vi "Make Default QPS.vi"() -> (3 "QPS settings":T1={"TWM pipe name"="", "meas"={"Measurement ID"=enum."Manual setup", "Description"="", "Switching matrix M"=[], "Signal frequency  (Hz)"=0.0, "Maximal signal amplitude (V)"=0.0, "PRs (samples)"=0, "PRe (samples)"=0, "MRs (samples)"=0, "MRe (samples)"=0, "Set PJVS frequency (Hz)"=0.0, "PJVS reference voltages (1 period, V)"=[], "Requiested PJVS steps"=0, "Sampling f (Hz)"=0.0, "Trigger mode"=enum."Trigger every MX switch", "Timing matrix (periods)"=[], "Record length (multiples of M)"=0, "Calculated"={"Triggers to next path (line of sequence)"=[], "Record samples"=0, "Sample indexes of switches"=[], "PRs (s)"=5.0, "PRe (s)"=5.0, "MRs (s)"=0.0, "MRe (s)"=0.0, "Trigger frequency  (Hz)"=0.0, "Measurement druation (s)"=0.0, "Samples per step"=0.0, "QPMX Sequence"=[], "PJVS segments frequency (Hz)"=50.0}, "No of required digitizers"=0, "No of required transducers"=0, "Transducer correction files"=[], "Digitizer correction file"=path "", "Algorithm"="TWM-PWRFFT", "plots_level"=1}, "PJVS setup"={"PJVS type"=enum."AC-supraVOLTcontrol", "Status Refnum"=refnum, "AC-supraVOLTcontrol"={"IP address:port (0.0.0.0:0000)"="", "Timeouts"={"TCP Read & Write (ms)"=0, "Sensors readout"=0, "PJVS setup"=0, "Nullmeter readout"=0, "Multiplexer setup"=0, "57XX setup"=0, "Generator setup"=0, "Synthesizer setup"=0, "Sampler readout"=0}, "Simulation mode"=FALSE, "Debug mode"=FALSE}, "NPL bias source"={"DataSocketCluster"={"Server Machine"="", "Client Machine"="", "Data"="", "TimeStamp"=0.0, "Count"=0, "Target Process"=""}}, "Manual PJVS"={"PJVS frequency (Hz)"=0.0, "Reference voltages (V)"=[], "File with PJVS voltages"=path ""}, "VTT PJVS"={"some VTT only property"=""}}, "Measurement status Ref"=refnum, "TWM status Ref"=refnum, "Abort Ref"=refnum, "AWG"={"AWG type"=enum."Agilent 331xxA to 332xxA", "FGEN Resource Name"="", "Source (Onboard Clock)"="", "FGEN Channel"="", "awg lib session"={"type"=enum."Agilent 331xxA to 332xxA", "VISA"="", "enable 10MHz ref"=FALSE, "cmi ckd2"={"VISA"="", "clock source"=enum."Auto", "manual ref clk"=FALSE, "ref clock [Hz]"=0.0, "div mode"=enum."Set divisor directly"}, "cmi sync v3"={"VISA"="", "baud rate [bd/s]"=0, "source"=enum."Auto", "hv range"=enum."10V", "fsrc is fixed"=FALSE, "fsrc [Hz]"=0.0, "freq integ [s]"=0.0, "freq filter"=0, "trig level"=enum."LVCMOS 3V3", "chn1 mode"=enum."Source divider", "chn1 level"=enum."Positive 3V3", "chn2 mode"=enum."Source divider", "chn2 level"=enum."Positive 3V3", "chn2 div"=0, "chn3 mode"=enum."Chn 1 Active", "chn3 level"=enum."Positive 3V3", "chn1 div entry"=enum."Set divisor directly", "chn1 dev limit [%]"=0.0, "chn1 check dev"=FALSE}, "trigger"={"source"=enum."Immediate", "level [V]"=0.0, "coupling"=enum."DC", "slope"=enum."POS"}, "HMF2500 cfg"={"Baud Rate"=0, "Parity"=0, "Data Bits"=0, "Flow Control"=0}}}} {"AWG"."awg lib session"."HMF2500 cfg"."Flow Control" items=["None", "XON/XOFF", "RTS/CTS", "XON/XOFF & RTS/CTS", "DTR/DSR", "XON/XOFF & DTR/DSR"]; "AWG"."awg lib session"."HMF2500 cfg"."Data Bits" items=["7"=7, "8"=8]; "AWG"."awg lib session"."HMF2500 cfg"."Parity" items=["None", "Odd", "Even", "Mark", "Space"]; "AWG"."awg lib session"."HMF2500 cfg"."Baud Rate" items=["300"=300, "600"=600, "1200"=1200, "2400"=2400, "4800"=4800, "9600"=9600, "19200"=19200]; "AWG"."awg lib session"."cmi sync v3"."chn2 div" min=1 max=100000000 step=1; "AWG"."awg lib session"."cmi sync v3"."fsrc [Hz]" format="%_8p"; "PJVS setup"."NPL bias source"."DataSocketCluster"."TimeStamp" format="%.2f"; "meas"."plots_level" max=4 step=1; "meas"."Calculated"."Trigger frequency  (Hz)" format="%#_6p"; "meas"."Record length (multiples of M)" min=1 step=1; "meas"."PJVS reference voltages (1 period, V)" format="%.9g"})   [LabVIEW 2020]
doc: "Returns QPS set to default values."
uses:
  General PJVS driver/QPSsettings.ctl
  Measurement/Type definitions/Measuement properties.ctl
  Measurement/Type definitions/Measurement ID.ctl
  Measurement/Type definitions/Trigger mode.ctl
  General PJVS driver/Type definitions/PJVS Setup.ctl
  General PJVS driver/Type definitions/PJVS Type.ctl
  PJVS drivers/acsvcontrol-driver/build/ACSVcontrol-driver_0.2.1.0.llb/Timeouts.ctl
  PJVS drivers/JV modified NPL Bias source/DataSocketCluster external.ctl
  General AWG/Type definitions/AWG.ctl
  General AWG/Type definitions/AWG type.ctl
  <instrlib>/niFgen/niFgen.llb/niFgen_ctl Sample Clock Source Values (Ring).ctl
  external libraries/AWG/AWG Session.ctl
  external libraries/AWG/AWG Type.ctl
  external libraries/AWG/CMI Clock Divider v2/CMI ckd2 Session.ctl
  external libraries/AWG/CMI Clock Divider v2/CMI ckd2 Source Mode.ctl
  external libraries/AWG/CMI Clock Divider v2/CMI ckd2 Divisor Mode.ctl
  external libraries/AWG/CMI Sync V3/CMI Sync V3 session.ctl
  external libraries/AWG/CMI Sync V3/Configure/CMI Sync V3 Reference Clock Source.ctl
  external libraries/AWG/CMI Sync V3/Configure/CMI Sync V3 HV input Range.ctl
  external libraries/AWG/CMI Sync V3/Configure/CMI Sync V3 Trigger Input Level.ctl
  external libraries/AWG/CMI Sync V3/Configure/CMI Sync V3 Channel 1 Mode.ctl
  external libraries/AWG/CMI Sync V3/Configure/CMI Sync V3 Channel Output Levels.ctl
  external libraries/AWG/CMI Sync V3/Configure/CMI Sync V3 Channel 2 Mode.ctl
  external libraries/AWG/CMI Sync V3/Configure/CMI Sync V3 Channel 3 Mode.ctl
  external libraries/AWG/CMI Sync V3/Configure/CMI Sync V3 Channel 1 Divisor Entry Mode.ctl
  external libraries/externals needed for AWG/ADC Trig Config.ctl
  external libraries/externals needed for AWG/ADC Trig Mode Source.ctl
  external libraries/externals needed for AWG/ADC Trig Coupling.ctl
  external libraries/externals needed for AWG/ADC Trig Slope.ctl
  external libraries/AWG/RaS HMF2500/HMF2500 Config.ctl
  external libraries/AWG/AWG.lvlib
  external libraries/AWG/CMI Sync V3/CMI Sync Unit V3.lvlib
  PJVS drivers/acsvcontrol-driver/build/ACSVcontrol-driver_0.2.1.0.llb/ACSVcontrol-driver.lvlib
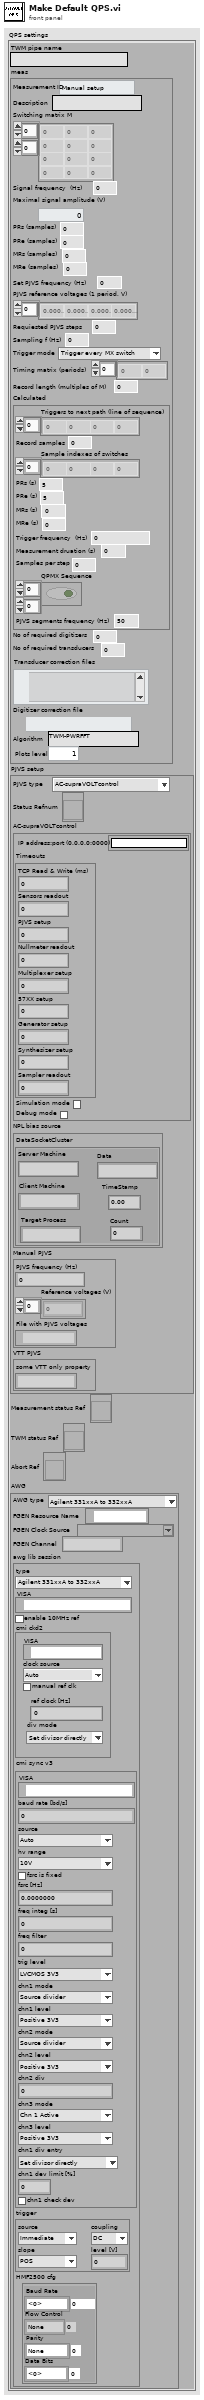
[diagram p1: front panel]
types:
  T1 = typedef "QPSsettings.ctl" = cluster{"TWM pipe name":string, "meas":T2, "PJVS setup":T5, "Measurement status Ref":refnum<vi>, "TWM status Ref":refnum<vi>, "Abort Ref":refnum<vi>, "AWG":T9}
  T2 = typedef "Measuement properties.ctl" = cluster{"Measurement ID":T3, "Description":string, "Switching matrix M":i32[][], "Signal frequency  (Hz)":dbl, "Maximal signal amplitude (V)":dbl, "PRs (samples)":u32, "PRe (samples)":u32, "MRs (samples)":u32, "MRe (samples)":u32, "Set PJVS frequency (Hz)":dbl, "PJVS reference voltages (1 period, V)":dbl[], "Requiested PJVS steps":u32, "Sampling f (Hz)":dbl, "Trigger mode":T4, "Timing matrix (periods)":i32[], "Record length (multiples of M)":u32, "Calculated":cluster{"Triggers to next path (line of sequence)":u32[], "Record samples":u32, "Sample indexes of switches":u32[], "PRs (s)":dbl, "PRe (s)":dbl, "MRs (s)":dbl, "MRe (s)":dbl, "Trigger frequency  (Hz)":dbl, "Measurement druation (s)":dbl, "Samples per step":dbl, "QPMX Sequence":bool[][], "PJVS segments frequency (Hz)":dbl}, "No of required digitizers":u32, "No of required transducers":u32, "Transducer correction files":path[], "Digitizer correction file":path, "Algorithm":string, "plots_level":u32}
  T3 = typedef "Measurement ID.ctl" = enum16{"Manual setup", "1 signal, 1 ADC, 1 PJVS", "1 phase (U, I), 1 ADC, 1 PJVS", "1 phase (U, I), 2 ADC, 1 PJVS", "1 phase (U, I), 3 ADC, 1 PJVS", "3 phases (U1..3, I1..3), 3 ADC, 1 PJVS"}
  T4 = typedef "Trigger mode.ctl" = enum16{"Trigger every MX switch", "Trigger every sample"}
  T5 = typedef "PJVS Setup.ctl" = cluster{"PJVS type":T6, "Status Refnum":refnum<vi>, "AC-supraVOLTcontrol":cluster{"IP address:port (0.0.0.0:0000)":string, "Timeouts":T7, "Simulation mode":bool, "Debug mode":bool}, "NPL bias source":cluster{"DataSocketCluster":T8}, "Manual PJVS":cluster{"PJVS frequency (Hz)":dbl, "Reference voltages (V)":dbl[], "File with PJVS voltages":path}, "VTT PJVS":cluster{"some VTT only property":string}}
  T6 = typedef "PJVS Type.ctl" = enum16{"AC-supraVOLTcontrol", "JV modified NPL bias control", "Manual PJVS", "VTT PJVS"}
  T7 = typedef "ACSVcontrol-driver.lvlib/Timeouts.ctl" = cluster{"TCP Read & Write (ms)":i32, "Sensors readout":i32, "PJVS setup":i32, "Nullmeter readout":i32, "Multiplexer setup":i32, "57XX setup":i32, "Generator setup":i32, "Synthesizer setup":i32, "Sampler readout":i32}
  T8 = typedef "DataSocketCluster external.ctl" = cluster{"Server Machine":string, "Client Machine":string, "Data":string, "TimeStamp":dbl, "Count":i32, "Target Process":string}
  T9 = typedef "AWG.ctl" = cluster{"AWG type":T10, "FGEN Resource Name":refnum<k15>, "Source (Onboard Clock)":T11, "FGEN Channel":string, "awg lib session":T12}
  T10 = typedef "AWG type.ctl" = enum16{"Agilent 331xxA to 332xxA", "Agilent 335xxA to 336xxA", "Tektronix AFG3101C", "R&S HMF25xx", "CMI Clock Divider v2", "CMI Sync Unit V3", "FGEN NI 5413", "Supracon PJVS Generator", "dummy"}
  T11 = typedef "niFgen_ctl Sample Clock Source Values (Ring).ctl" = string
  T12 = typedef "AWG.lvlib/AWG Session.ctl" = cluster{"type":T13, "VISA":refnum<visa-resource-name>, "enable 10MHz ref":bool, "cmi ckd2":T14, "cmi sync v3":T17, "trigger":T26, "HMF2500 cfg":T30}
  T13 = typedef "AWG.lvlib/AWG Type.ctl" = enum16{"Agilent 331xxA to 332xxA", "Agilent 335xxA to 336xxA", "Tektronix AFG3101C", "R&S HMF25xx", "CMI Clock Divider v2", "CMI Sync Unit V3", "dummy"}
  T14 = typedef "AWG.lvlib/CMI ckd2 Session.ctl" = cluster{"VISA":refnum<visa-resource-name>, "clock source":T15, "manual ref clk":bool, "ref clock [Hz]":dbl, "div mode":T16}
  T15 = typedef "AWG.lvlib/CMI ckd2 Source Mode.ctl" = enum16{"Auto", "LF clock", "HF clock", "Internal"}
  T16 = typedef "AWG.lvlib/CMI ckd2 Divisor Mode.ctl" = enum16{"Set divisor directly", "Set divisor by frequency"}
  T17 = typedef "AWG.lvlib/CMI Sync Unit V3.lvlib/CMI Sync V3 session.ctl" = cluster{"VISA":refnum<visa-resource-name>, "baud rate [bd/s]":i32, "source":T18, "hv range":T19, "fsrc is fixed":bool, "fsrc [Hz]":dbl, "freq integ [s]":dbl, "freq filter":i32, "trig level":T20, "chn1 mode":T21, "chn1 level":T22, "chn2 mode":T23, "chn2 level":T22, "chn2 div":i32, "chn3 mode":T24, "chn3 level":T22, "chn1 div entry":T25, "chn1 dev limit [%]":dbl, "chn1 check dev":bool}
  T18 = typedef "AWG.lvlib/CMI Sync Unit V3.lvlib/CMI Sync V3 Reference Clock Source.ctl" = enum16{"Auto", "Internal", "Logic", "Sine", "HV"}
  T19 = typedef "AWG.lvlib/CMI Sync Unit V3.lvlib/CMI Sync V3 HV input Range.ctl" = enum16{"10V", "60V", "250V", "1kV"}
  T20 = typedef "AWG.lvlib/CMI Sync Unit V3.lvlib/CMI Sync V3 Trigger Input Level.ctl" = enum16{"LVCMOS 3V3", "TTL 5V"}
  T21 = typedef "AWG.lvlib/CMI Sync Unit V3.lvlib/CMI Sync V3 Channel 1 Mode.ctl" = enum16{"Source divider", "DDS absolute", "DDS ratio", "DDS ratio M/N"}
  T22 = typedef "AWG.lvlib/CMI Sync Unit V3.lvlib/CMI Sync V3 Channel Output Levels.ctl" = enum16{"Positive 3V3", "Negative 3V3", "Positive 5V", "Negative 5V"}
  T23 = typedef "AWG.lvlib/CMI Sync Unit V3.lvlib/CMI Sync V3 Channel 2 Mode.ctl" = enum16{"Source divider", "Chn 1 divide"}
  T24 = typedef "AWG.lvlib/CMI Sync Unit V3.lvlib/CMI Sync V3 Channel 3 Mode.ctl" = enum16{"Chn 1 Active", "Chn 2 Active", "Chn 1 Trigger", "Chn 2 Trigger", "Gate", "PPS", "10MHz"}
  T25 = typedef "AWG.lvlib/CMI Sync Unit V3.lvlib/CMI Sync V3 Channel 1 Divisor Entry Mode.ctl" = enum16{"Set divisor directly", "Calculate nearest divisor from measured fx"}
  T26 = typedef "ADC Trig Config.ctl" = cluster{"source":T27, "level [V]":dbl, "coupling":T28, "slope":T29}
  T27 = typedef "ADC Trig Mode Source.ctl" = enum16{"Immediate", "External", "Level"}
  T28 = typedef "ADC Trig Coupling.ctl" = enum16{"DC", "AC"}
  T29 = typedef "ADC Trig Slope.ctl" = enum16{"POS", "NEG"}
  T30 = typedef "AWG.lvlib/HMF2500 Config.ctl" = cluster{"Baud Rate":u32, "Parity":u16, "Data Bits":u16, "Flow Control":u16}
  T31 = cluster{"Triggers to next path (line of sequence)":u32[], "Record samples":u32, "Sample indexes of switches":u32[], "PRs (s)":dbl, "PRe (s)":dbl, "MRs (s)":dbl, "MRe (s)":dbl, "Trigger frequency  (Hz)":dbl, "Measurement druation (s)":dbl, "Samples per step":dbl, "QPMX Sequence":bool[][], "PJVS segments frequency (Hz)":dbl}
  T32 = cluster{"PJVS frequency (Hz)":dbl, "Reference voltages (V)":dbl[], "File with PJVS voltages":path}
  T33 = cluster{"IP address:port (0.0.0.0:0000)":string, "Timeouts":T7, "Simulation mode":bool, "Debug mode":bool}
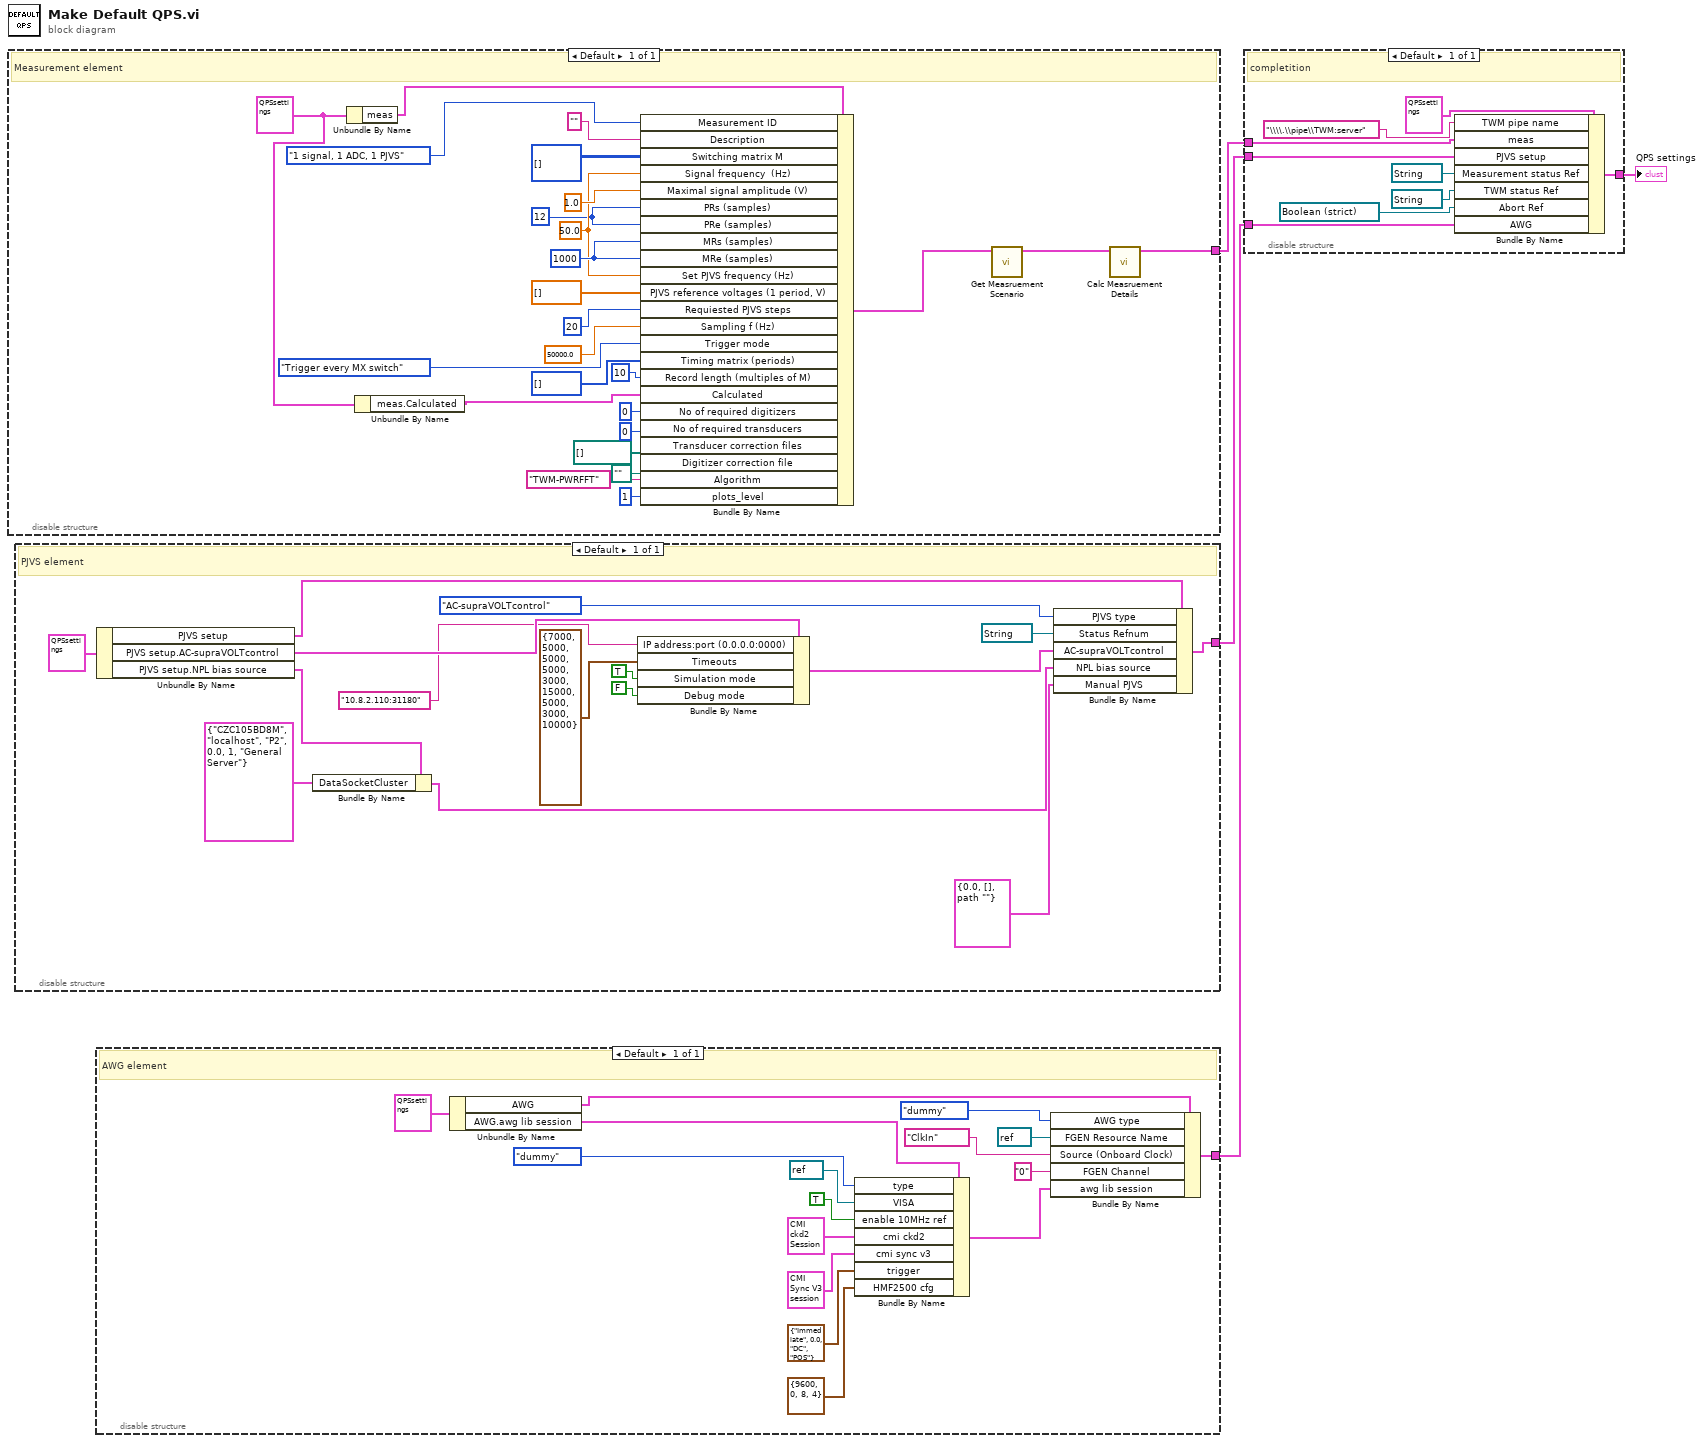
[diagram p0: block diagram]
diagram:
  n1 = disable-structure shown="Default" {
    disable-tunnel: [w16] -> w3
    frame Enabled {
      w7 = u32 12 ("Signal frequency  (Hz)")
      w9 = T1 {"TWM pipe name"="\\\\.\\pipe\\TWM:server", "meas"={"Measurement ID"=enum."1 signal, 1 ADC, 1 PJVS", "Description"="3 phase, 3 ADC, 1 PJVS", "Switching matrix M"=[], "Signal frequency  (Hz)"=50.0, "Maximal signal amplitude (V)"=0.0, "PRs (samples)"=1, "PRe (samples)"=10, "MRs (samples)"=0, "MRe (samples)"=0, "Set PJVS frequency (Hz)"=50.0, "PJVS reference voltages (1 period, V)"=[], "Requiested PJVS steps"=10, "Sampling f (Hz)"=7000.0, "Trigger mode"=enum."Trigger every MX switch", "Timing matrix (periods)"=[], "Record length (multiples of M)"=1, "Calculated"={"Triggers to next path (line of sequence)"=[], "Record samples"=0, "Sample indexes of switches"=[], "PRs (s)"=0.0, "PRe (s)"=0.0, "MRs (s)"=0.0, "MRe (s)"=0.0, "Trigger frequency  (Hz)"=50.0, "Measurement druation (s)"=0.0, "Samples per step"=0.0, "QPMX Sequence"=[], "PJVS segments frequency (Hz)"=50.0}, "No of required digitizers"=0, "No of required transducers"=0, "Transducer correction files"=[], "Digitizer correction file"=path "", "Algorithm"="TWM-PWRFFT", "plots_level"=1}, "PJVS setup"={"PJVS type"=enum."AC-supraVOLTcontrol", "Status Refnum"=refnum, "AC-supraVOLTcontrol"={"IP address:port (0.0.0.0:0000)"="0.0.0.0:0000", "Timeouts"={"TCP Read & Write (ms)"=7000, "Sensors readout"=5000, "PJVS setup"=10000, "Nullmeter readout"=5000, "Multiplexer setup"=3000, "57XX setup"=15000, "Generator setup"=5000, "Synthesizer setup"=3000, "Sampler readout"=10000}, "Simulation mode"=FALSE, "Debug mode"=FALSE}, "NPL bias source"={"DataSocketCluster"={"Server Machine"="CZC105BD8M", "Client Machine"="localhost", "Data"="P2", "TimeStamp"=0.0, "Count"=1, "Target Process"="General Server"}}, "Manual PJVS"={"PJVS frequency (Hz)"=0.0, "Reference voltages (V)"=[], "File with PJVS voltages"=path ""}, "VTT PJVS"={"some VTT only property"=""}}, "Measurement status Ref"=refnum, "TWM status Ref"=refnum, "Abort Ref"=refnum, "AWG"={"AWG type"=enum."Agilent 331xxA to 332xxA", "FGEN Resource Name"="", "Source (Onboard Clock)"="OnboardClock", "FGEN Channel"="0", "awg lib session"={"type"=enum."Agilent 331xxA to 332xxA", "VISA"="", "enable 10MHz ref"=FALSE, "cmi ckd2"={"VISA"="", "clock source"=enum."Auto", "manual ref clk"=FALSE, "ref clock [Hz]"=0.0, "div mode"=enum."Set divisor directly"}, "cmi sync v3"={"VISA"="", "baud rate [bd/s]"=115200, "source"=enum."Auto", "hv range"=enum."1kV", "fsrc is fixed"=FALSE, "fsrc [Hz]"=10000000.0, "freq integ [s]"=1.0, "freq filter"=5, "trig level"=enum."TTL 5V", "chn1 mode"=enum."Source divider", "chn1 level"=enum."Positive 5V", "chn2 mode"=enum."Source divider", "chn2 level"=enum."Positive 5V", "chn2 div"=1, "chn3 mode"=enum."Chn 1 Active", "chn3 level"=enum."Positive 5V", "chn1 div entry"=enum."Calculate nearest divisor from measured fx", "chn1 dev limit [%]"=1.0, "chn1 check dev"=FALSE}, "trigger"={"source"=enum."Immediate", "level [V]"=0.0, "coupling"=enum."DC", "slope"=enum."POS"}, "HMF2500 cfg"={"Baud Rate"=9600, "Parity"=0, "Data Bits"=8, "Flow Control"=4}}}} ("QPS settings")
      w25 = u32 1000 ("PRs (s)")
      w24 = 50.0 ("Signal frequency  (Hz)")
      # "Measurement element"
      n2 = Unbundle By Name(w9) -> ("meas"=w29:T2)
      n3 = Unbundle By Name(w9) -> ("meas.Calculated"=w8:T31)
      n4 = Bundle By Name(cluster=w29, "Measurement ID"=Measurement_ID."1 signal, 1 ADC, 1 PJVS", "Description"="", "Switching matrix M"=u32[][] [], "Signal frequency  (Hz)"=w24, "Maximal signal amplitude (V)"=1.0, "PRs (samples)"=w7, "PRe (samples)"=w7, "MRs (samples)"=w25, "MRe (samples)"=w25, "Set PJVS frequency (Hz)"=w24, "PJVS reference voltages (1 period, V)"=dbl[] [], "Requiested PJVS steps"=u32 20, "Sampling f (Hz)"=50000.0, "Trigger mode"=Trigger_mode."Trigger every MX switch", "Timing matrix (periods)"=i32[] [], "Record length (multiples of M)"=u32 10, "Calculated"=w8, "No of required digitizers"=u32 0, "No of required transducers"=u32 0, "Transducer correction files"=path[] [], "Digitizer correction file"=path "", "Algorithm"="TWM-PWRFFT", "plots_level"=u32 1) -> (w17:T2)
      n5 = call "Get Measruement Scenario.vi"("Measurement properties"=w17) -> ("Measurement properties out"=w27:T2)  [unwired: 10 in]
      n6 = call "Calc Measruement Details.vi"("Measurement properties"=w27) -> ("Measurement properties out"=w16:T2)  [unwired: 10 in]
    }
  }
  n7 = disable-structure shown="Default" {
    disable-tunnel: [w32] -> w2
    frame Enabled {
      # "PJVS element"
      n8 = Unbundle By Name(T1 {"TWM pipe name"="\\\\.\\pipe\\TWM:server", "meas"={"Measurement ID"=enum."1 signal, 1 ADC, 1 PJVS", "Description"="3 phase, 3 ADC, 1 PJVS", "Switching matrix M"=[], "Signal frequency  (Hz)"=50.0, "Maximal signal amplitude (V)"=0.0, "PRs (samples)"=1, "PRe (samples)"=10, "MRs (samples)"=0, "MRe (samples)"=0, "Set PJVS frequency (Hz)"=50.0, "PJVS reference voltages (1 period, V)"=[], "Requiested PJVS steps"=10, "Sampling f (Hz)"=7000.0, "Trigger mode"=enum."Trigger every MX switch", "Timing matrix (periods)"=[], "Record length (multiples of M)"=1, "Calculated"={"Triggers to next path (line of sequence)"=[], "Record samples"=0, "Sample indexes of switches"=[], "PRs (s)"=0.0, "PRe (s)"=0.0, "MRs (s)"=0.0, "MRe (s)"=0.0, "Trigger frequency  (Hz)"=50.0, "Measurement druation (s)"=0.0, "Samples per step"=0.0, "QPMX Sequence"=[], "PJVS segments frequency (Hz)"=50.0}, "No of required digitizers"=0, "No of required transducers"=0, "Transducer correction files"=[], "Digitizer correction file"=path "", "Algorithm"="TWM-PWRFFT", "plots_level"=1}, "PJVS setup"={"PJVS type"=enum."AC-supraVOLTcontrol", "Status Refnum"=refnum, "AC-supraVOLTcontrol"={"IP address:port (0.0.0.0:0000)"="0.0.0.0:0000", "Timeouts"={"TCP Read & Write (ms)"=7000, "Sensors readout"=5000, "PJVS setup"=10000, "Nullmeter readout"=5000, "Multiplexer setup"=3000, "57XX setup"=15000, "Generator setup"=5000, "Synthesizer setup"=3000, "Sampler readout"=10000}, "Simulation mode"=FALSE, "Debug mode"=FALSE}, "NPL bias source"={"DataSocketCluster"={"Server Machine"="CZC105BD8M", "Client Machine"="localhost", "Data"="P2", "TimeStamp"=0.0, "Count"=1, "Target Process"="General Server"}}, "Manual PJVS"={"PJVS frequency (Hz)"=0.0, "Reference voltages (V)"=[], "File with PJVS voltages"=path ""}, "VTT PJVS"={"some VTT only property"=""}}, "Measurement status Ref"=refnum, "TWM status Ref"=refnum, "Abort Ref"=refnum, "AWG"={"AWG type"=enum."Agilent 331xxA to 332xxA", "FGEN Resource Name"="", "Source (Onboard Clock)"="OnboardClock", "FGEN Channel"="0", "awg lib session"={"type"=enum."Agilent 331xxA to 332xxA", "VISA"="", "enable 10MHz ref"=FALSE, "cmi ckd2"={"VISA"="", "clock source"=enum."Auto", "manual ref clk"=FALSE, "ref clock [Hz]"=0.0, "div mode"=enum."Set divisor directly"}, "cmi sync v3"={"VISA"="", "baud rate [bd/s]"=115200, "source"=enum."Auto", "hv range"=enum."1kV", "fsrc is fixed"=FALSE, "fsrc [Hz]"=10000000.0, "freq integ [s]"=1.0, "freq filter"=5, "trig level"=enum."TTL 5V", "chn1 mode"=enum."Source divider", "chn1 level"=enum."Positive 5V", "chn2 mode"=enum."Source divider", "chn2 level"=enum."Positive 5V", "chn2 div"=1, "chn3 mode"=enum."Chn 1 Active", "chn3 level"=enum."Positive 5V", "chn1 div entry"=enum."Calculate nearest divisor from measured fx", "chn1 dev limit [%]"=1.0, "chn1 check dev"=FALSE}, "trigger"={"source"=enum."Immediate", "level [V]"=0.0, "coupling"=enum."DC", "slope"=enum."POS"}, "HMF2500 cfg"={"Baud Rate"=9600, "Parity"=0, "Data Bits"=8, "Flow Control"=4}}}} ("QPS settings")) -> ("PJVS setup"=w44:T5, "PJVS setup.AC-supraVOLTcontrol"=w41:T33, "PJVS setup.NPL bias source"=w35:cluster{"DataSocketCluster":T8})
      n9 = Bundle By Name(cluster=w35, "DataSocketCluster"=T8 {"Server Machine"="CZC105BD8M", "Client Machine"="localhost", "Data"="P2", "TimeStamp"=0.0, "Count"=1, "Target Process"="General Server"}) -> (w34:cluster{"DataSocketCluster":T8})
      n10 = Bundle By Name(cluster=w41, "IP address:port (0.0.0.0:0000)"="10.8.2.110:31180", "Timeouts"=T7 {"TCP Read & Write (ms)"=7000, "Sensors readout"=5000, "PJVS setup"=5000, "Nullmeter readout"=5000, "Multiplexer setup"=3000, "57XX setup"=15000, "Generator setup"=5000, "Synthesizer setup"=3000, "Sampler readout"=10000}, "Simulation mode"=TRUE, "Debug mode"=FALSE) -> (w40:T33)
      n11 = Bundle By Name(cluster=w44, "PJVS type"=PJVS_Type."AC-supraVOLTcontrol", "Status Refnum"=refnum<vi> refnum, "AC-supraVOLTcontrol"=w40, "NPL bias source"=w34, "Manual PJVS"=T32 {"PJVS frequency (Hz)"=0.0, "Reference voltages (V)"=[], "File with PJVS voltages"=path ""}) -> (w32:T5)
    }
  }
  n12 = disable-structure shown="Default" {
    disable-tunnel: [w46] -> w1
    frame Enabled {
      # "AWG element"
      n13 = Unbundle By Name(T1 {"TWM pipe name"="\\\\.\\pipe\\TWM:server", "meas"={"Measurement ID"=enum."1 signal, 1 ADC, 1 PJVS", "Description"="3 phase, 3 ADC, 1 PJVS", "Switching matrix M"=[], "Signal frequency  (Hz)"=50.0, "Maximal signal amplitude (V)"=0.0, "PRs (samples)"=1, "PRe (samples)"=10, "MRs (samples)"=0, "MRe (samples)"=0, "Set PJVS frequency (Hz)"=50.0, "PJVS reference voltages (1 period, V)"=[], "Requiested PJVS steps"=10, "Sampling f (Hz)"=7000.0, "Trigger mode"=enum."Trigger every MX switch", "Timing matrix (periods)"=[], "Record length (multiples of M)"=1, "Calculated"={"Triggers to next path (line of sequence)"=[], "Record samples"=0, "Sample indexes of switches"=[], "PRs (s)"=0.0, "PRe (s)"=0.0, "MRs (s)"=0.0, "MRe (s)"=0.0, "Trigger frequency  (Hz)"=50.0, "Measurement druation (s)"=0.0, "Samples per step"=0.0, "QPMX Sequence"=[], "PJVS segments frequency (Hz)"=50.0}, "No of required digitizers"=0, "No of required transducers"=0, "Transducer correction files"=[], "Digitizer correction file"=path "", "Algorithm"="TWM-PWRFFT", "plots_level"=1}, "PJVS setup"={"PJVS type"=enum."AC-supraVOLTcontrol", "Status Refnum"=refnum, "AC-supraVOLTcontrol"={"IP address:port (0.0.0.0:0000)"="0.0.0.0:0000", "Timeouts"={"TCP Read & Write (ms)"=7000, "Sensors readout"=5000, "PJVS setup"=10000, "Nullmeter readout"=5000, "Multiplexer setup"=3000, "57XX setup"=15000, "Generator setup"=5000, "Synthesizer setup"=3000, "Sampler readout"=10000}, "Simulation mode"=FALSE, "Debug mode"=FALSE}, "NPL bias source"={"DataSocketCluster"={"Server Machine"="CZC105BD8M", "Client Machine"="localhost", "Data"="P2", "TimeStamp"=0.0, "Count"=1, "Target Process"="General Server"}}, "Manual PJVS"={"PJVS frequency (Hz)"=0.0, "Reference voltages (V)"=[], "File with PJVS voltages"=path ""}, "VTT PJVS"={"some VTT only property"=""}}, "Measurement status Ref"=refnum, "TWM status Ref"=refnum, "Abort Ref"=refnum, "AWG"={"AWG type"=enum."Agilent 331xxA to 332xxA", "FGEN Resource Name"="", "Source (Onboard Clock)"="OnboardClock", "FGEN Channel"="0", "awg lib session"={"type"=enum."Agilent 331xxA to 332xxA", "VISA"="", "enable 10MHz ref"=FALSE, "cmi ckd2"={"VISA"="", "clock source"=enum."Auto", "manual ref clk"=FALSE, "ref clock [Hz]"=0.0, "div mode"=enum."Set divisor directly"}, "cmi sync v3"={"VISA"="", "baud rate [bd/s]"=115200, "source"=enum."Auto", "hv range"=enum."1kV", "fsrc is fixed"=FALSE, "fsrc [Hz]"=10000000.0, "freq integ [s]"=1.0, "freq filter"=5, "trig level"=enum."TTL 5V", "chn1 mode"=enum."Source divider", "chn1 level"=enum."Positive 5V", "chn2 mode"=enum."Source divider", "chn2 level"=enum."Positive 5V", "chn2 div"=1, "chn3 mode"=enum."Chn 1 Active", "chn3 level"=enum."Positive 5V", "chn1 div entry"=enum."Calculate nearest divisor from measured fx", "chn1 dev limit [%]"=1.0, "chn1 check dev"=FALSE}, "trigger"={"source"=enum."Immediate", "level [V]"=0.0, "coupling"=enum."DC", "slope"=enum."POS"}, "HMF2500 cfg"={"Baud Rate"=9600, "Parity"=0, "Data Bits"=8, "Flow Control"=4}}}} ("QPS settings")) -> ("AWG"=w60:T9, "AWG.awg lib session"=w55:T12)
      n14 = Bundle By Name(cluster=w55, "type"=AWG_Type."dummy", "VISA"=refnum<visa-resource-name> refnum, "enable 10MHz ref"=TRUE, "cmi ckd2"=T14 {"VISA"="", "clock source"=enum."Auto", "manual ref clk"=FALSE, "ref clock [Hz]"=0.0, "div mode"=enum."Set divisor directly"}, "cmi sync v3"=T17 {"VISA"="", "baud rate [bd/s]"=115200, "source"=enum."Auto", "hv range"=enum."1kV", "fsrc is fixed"=FALSE, "fsrc [Hz]"=10000000.0, "freq integ [s]"=1.0, "freq filter"=5, "trig level"=enum."TTL 5V", "chn1 mode"=enum."Source divider", "chn1 level"=enum."Positive 5V", "chn2 mode"=enum."Source divider", "chn2 level"=enum."Positive 5V", "chn2 div"=1, "chn3 mode"=enum."Chn 1 Active", "chn3 level"=enum."Positive 5V", "chn1 div entry"=enum."Calculate nearest divisor from measured fx", "chn1 dev limit [%]"=1.0, "chn1 check dev"=FALSE}, "trigger"=T26 {"source"=enum."Immediate", "level [V]"=0.0, "coupling"=enum."DC", "slope"=enum."POS"}, "HMF2500 cfg"=T30 {"Baud Rate"=9600, "Parity"=0, "Data Bits"=8, "Flow Control"=4}) -> (w47:T12)
      n15 = Bundle By Name(cluster=w60, "AWG type"=AWG_type."dummy", "FGEN Resource Name"=refnum<k15> refnum, "Source (Onboard Clock)"=T11 "ClkIn", "FGEN Channel"="0", "awg lib session"=w47) -> (w46:T9)
    }
  }
  n16 = disable-structure shown="Default" {
    disable-tunnel: [w69] -> w4
    disable-tunnel: w3 -> [w64]
    disable-tunnel: w2 -> [w63]
    disable-tunnel: w1 -> [w62]
    frame Enabled {
      # "completition"
      n17 = Bundle By Name(cluster=T1 {"TWM pipe name"="\\\\.\\pipe\\TWM:server", "meas"={"Measurement ID"=enum."1 signal, 1 ADC, 1 PJVS", "Description"="3 phase, 3 ADC, 1 PJVS", "Switching matrix M"=[], "Signal frequency  (Hz)"=50.0, "Maximal signal amplitude (V)"=0.0, "PRs (samples)"=1, "PRe (samples)"=10, "MRs (samples)"=0, "MRe (samples)"=0, "Set PJVS frequency (Hz)"=50.0, "PJVS reference voltages (1 period, V)"=[], "Requiested PJVS steps"=10, "Sampling f (Hz)"=7000.0, "Trigger mode"=enum."Trigger every MX switch", "Timing matrix (periods)"=[], "Record length (multiples of M)"=1, "Calculated"={"Triggers to next path (line of sequence)"=[], "Record samples"=0, "Sample indexes of switches"=[], "PRs (s)"=0.0, "PRe (s)"=0.0, "MRs (s)"=0.0, "MRe (s)"=0.0, "Trigger frequency  (Hz)"=50.0, "Measurement druation (s)"=0.0, "Samples per step"=0.0, "QPMX Sequence"=[], "PJVS segments frequency (Hz)"=50.0}, "No of required digitizers"=0, "No of required transducers"=0, "Transducer correction files"=[], "Digitizer correction file"=path "", "Algorithm"="TWM-PWRFFT", "plots_level"=1}, "PJVS setup"={"PJVS type"=enum."AC-supraVOLTcontrol", "Status Refnum"=refnum, "AC-supraVOLTcontrol"={"IP address:port (0.0.0.0:0000)"="0.0.0.0:0000", "Timeouts"={"TCP Read & Write (ms)"=7000, "Sensors readout"=5000, "PJVS setup"=10000, "Nullmeter readout"=5000, "Multiplexer setup"=3000, "57XX setup"=15000, "Generator setup"=5000, "Synthesizer setup"=3000, "Sampler readout"=10000}, "Simulation mode"=FALSE, "Debug mode"=FALSE}, "NPL bias source"={"DataSocketCluster"={"Server Machine"="CZC105BD8M", "Client Machine"="localhost", "Data"="P2", "TimeStamp"=0.0, "Count"=1, "Target Process"="General Server"}}, "Manual PJVS"={"PJVS frequency (Hz)"=0.0, "Reference voltages (V)"=[], "File with PJVS voltages"=path ""}, "VTT PJVS"={"some VTT only property"=""}}, "Measurement status Ref"=refnum, "TWM status Ref"=refnum, "Abort Ref"=refnum, "AWG"={"AWG type"=enum."Agilent 331xxA to 332xxA", "FGEN Resource Name"="", "Source (Onboard Clock)"="OnboardClock", "FGEN Channel"="0", "awg lib session"={"type"=enum."Agilent 331xxA to 332xxA", "VISA"="", "enable 10MHz ref"=FALSE, "cmi ckd2"={"VISA"="", "clock source"=enum."Auto", "manual ref clk"=FALSE, "ref clock [Hz]"=0.0, "div mode"=enum."Set divisor directly"}, "cmi sync v3"={"VISA"="", "baud rate [bd/s]"=115200, "source"=enum."Auto", "hv range"=enum."1kV", "fsrc is fixed"=FALSE, "fsrc [Hz]"=10000000.0, "freq integ [s]"=1.0, "freq filter"=5, "trig level"=enum."TTL 5V", "chn1 mode"=enum."Source divider", "chn1 level"=enum."Positive 5V", "chn2 mode"=enum."Source divider", "chn2 level"=enum."Positive 5V", "chn2 div"=1, "chn3 mode"=enum."Chn 1 Active", "chn3 level"=enum."Positive 5V", "chn1 div entry"=enum."Calculate nearest divisor from measured fx", "chn1 dev limit [%]"=1.0, "chn1 check dev"=FALSE}, "trigger"={"source"=enum."Immediate", "level [V]"=0.0, "coupling"=enum."DC", "slope"=enum."POS"}, "HMF2500 cfg"={"Baud Rate"=9600, "Parity"=0, "Data Bits"=8, "Flow Control"=4}}}} ("QPS settings"), "TWM pipe name"="\\\\.\\pipe\\TWM:server", "meas"=w64, "PJVS setup"=w63, "Measurement status Ref"=refnum<vi> refnum, "TWM status Ref"=refnum<vi> refnum, "Abort Ref"=refnum<vi> refnum, "AWG"=w62) -> (w69:T1)
    }
  }
  "QPS settings" <- w4
